vi "Rename Tags in Project File.vi"(8 "error in (no error)":errorcluster, 10 "Rename Tags[]":T1[](array[typedef]), 11 "Project Path":path) -> (0 "error out":errorcluster, 3 "Project Path Out":path)   [LabVIEW 2016, in "SLL Scripting.lvlib"]
doc: "Renames the identified tags in Project file with the user specified tag values in fields like Build Specification Name, Build Output Location, Company Name and any other string fields present in the Project file.\n\nSince this VI basically just does a string match and replace, care needs to be taken to ensure that the tag names would be unique and won't conflict with rest of text/fields.\n\nOne suggested way of naming the tags is [%TAG_NAME%]"
uses:
  SLL Scripting.lvlib
  _Typedefs/Rename Item Cluster.ctl
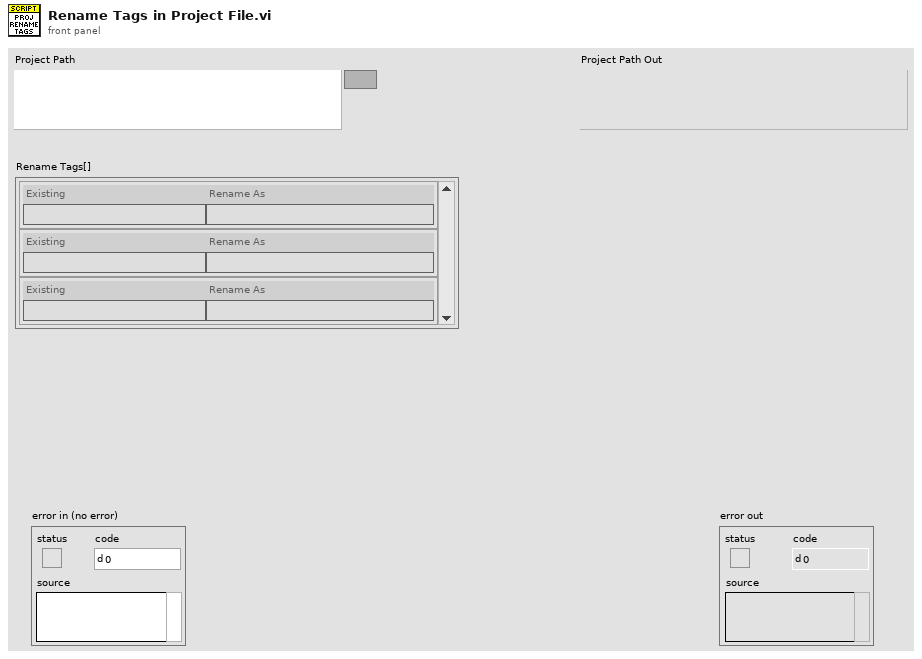
[diagram p1: front panel]
types:
  T1 = typedef "SLL Scripting.lvlib/Rename Item Cluster.ctl" = cluster{"Existing":string, "Rename As":string}
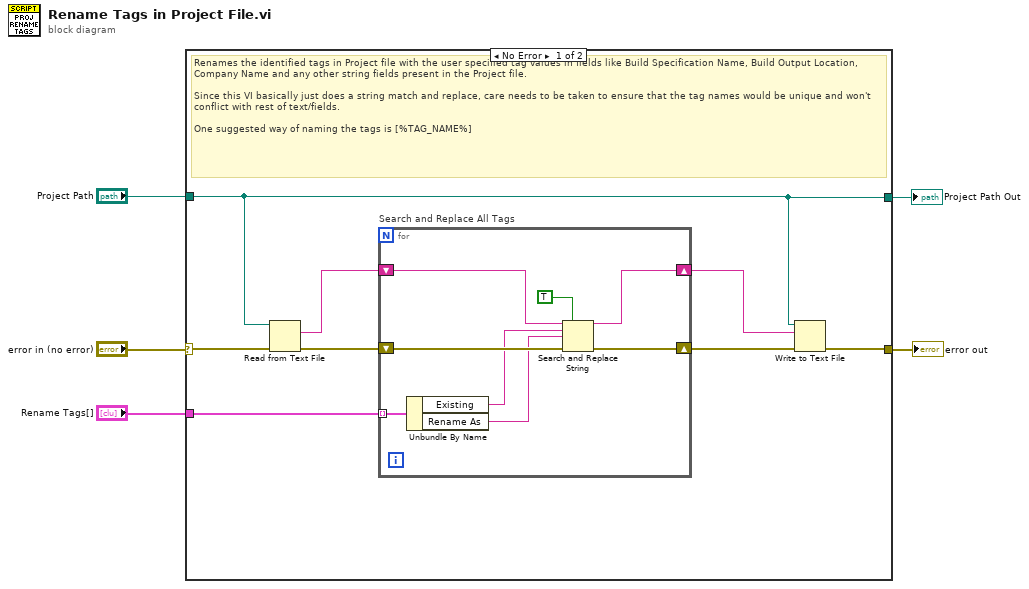
[diagram p0: block diagram]
diagram:
  n1 = case shown="No Error" "error in (no error)" {
    selector: "error in (no error)" -> [w13 w23]
    tunnel: [w8 w23] -> w4
    tunnel: "Project Path" -> [w6 w22]
    tunnel: "Rename Tags[]" -> [w10 _]
    tunnel: [w6 w22] -> w1
    frame No Error {
      # "Renames the identified tags in Project file with the user specified tag values in fields like Build Specification Name, Build Output Location, Company Name and any other string fields present in the Project file.\n\nSince this VI basically just does a string match and replace, care needs to be taken to ensure that the tag names would be unique and won't conflict with rest of text/fields.\n\nOne suggested way of naming the tags is [%TAG_NAME%]"
      n2 = Read from Text File(file (use dialog)=w6, error in=w13) -> (text=w9:string, error out=w12:errorcluster)  [unwired: 2 in, 2 out]
      n3 = for "Search and Replace All Tags" {
        shift-right: [w20] -> w11
        shift-left: w12 -> [w21]
        tunnel: w10 -> [w19] mode=indexing
        shift-right: [w17] -> w7
        shift-left: w9 -> [w18]
        n4 = Unbundle By Name(w19) -> ("Existing"=w15:string, "Rename As"=w14:string)
        n5 = Search and Replace String(replace all?=TRUE ("replace all? (F)"), input string=w18, search string=w15, replace string=w14, error in=w21) -> (result string=w17:string, error out=w20:errorcluster)  [unwired: 3 in, 2 out]
      }
      n6 = Write to Text File(file (use dialog)=w6, text=w7, error in=w11) -> (error out=w8:errorcluster)  [unwired: 1 in, 2 out]
    }
    frame Error {
    }
  }
  "error out" <- w4
  "Project Path Out" <- w1
